vi "External Caller.vi"() -> ()   [LabVIEW 2024]
uses:
  Libraries/Clon/Clon.lvlib
panel:
  in  "Refresh Button":bool
  out "Already running?":bool
  out "Status":string
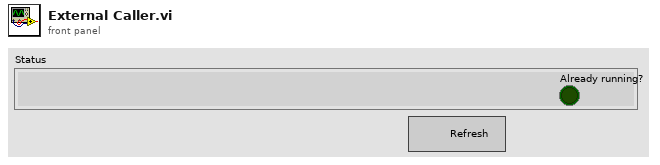
[diagram p1: front panel]
types:
  T1 = typedef "Clon.lvlib/Broadcast Events--cluster.ctl" = cluster{"Module Did Init":refnum<user-event>, "Status Updated":refnum<user-event>, "Error Reported":refnum<user-event>, "Did Something":refnum<user-event>, "Module Did Stop":refnum<user-event>, "Update Module Execution Status":refnum<user-event>}
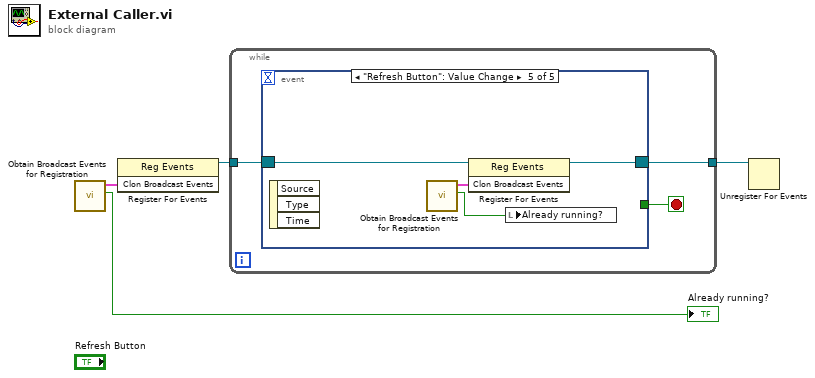
[diagram p0: block diagram]
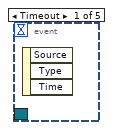
[diagram p2: hidden frame]
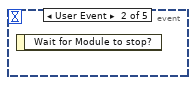
[diagram p3: hidden frame]
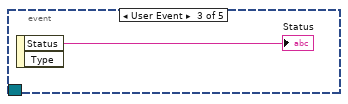
[diagram p4: hidden frame]
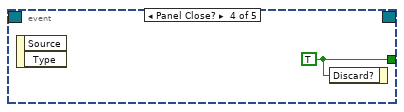
[diagram p5: hidden frame]
diagram:
  n1 = call "Obtain Broadcast Events for Registration.vi"() -> ("Already running?"=→"Already running?":bool, "Clon Broadcast Events"=w4:T1)  [unwired: 9 in, 1 out]
  n2 = register-events(w4) -> (reference out=w3:refnum<event-registration>)  [unwired: 2 in, 1 out]
  n3 = while {
    tunnel: w3 -> [w7]
    tunnel: [w6] -> w2
    stop <- w5 stop-if-true
    n4 = event shown="[4] \"Refresh Button\": Value Change" {
      selector: w7 -> [_ _ _ _ w12]
      dyn-events: [_ _ _ _ w11] -> w6
      timeout: _ -> [_ _ _ _ _]
      tunnel: [_ _ _ w9 _] -> w5
      event Timeout {
        n5 = event-data() -> ()  [unwired: 1 in, 3 out]
      }
      event User Event {
        n6 = event-data() -> ()  [unwired: 1 in, 1 out]
      }
      event User Event {
        n7 = event-data() -> ("Status"=→"Status":string)  [unwired: 1 in, 1 out]
      }
      event Panel Close? {
        w9 = TRUE ("Discard?")
        n8 = event-data() -> ()  [unwired: 1 in, 2 out]
        n9 = event-data("Discard?"=w9) -> ()  [unwired: 1 in, 1 out]
      }
      event "Refresh Button": Value Change {
        n10 = event-data() -> ()  [unwired: 1 in, 3 out]
        n11 = call "Obtain Broadcast Events for Registration.vi"() -> ("Already running?"=w10:bool, "Clon Broadcast Events"=w13:T1)  [unwired: 9 in, 1 out]
        n12 = register-events(reference=w12, w13) -> (reference out=w11:refnum<event-registration>)  [unwired: 1 in, 1 out]
        n13 = local write "Already running?"(w10) -> ()
      }
    }
  }
  n14 = Unregister For Events(event registration refnum=w2) -> ()  [unwired: 1 in, 1 out]
